vi "Write 16bit Wave.vi"() -> ()   [LabVIEW 2020]
uses:
  <vilib>/Analysis/NI_AALBase.lvlib
panel:
  out "16bit integer":i16[](array[numeric])
  # "ssh_init: Network error: Cannot assign requested address"
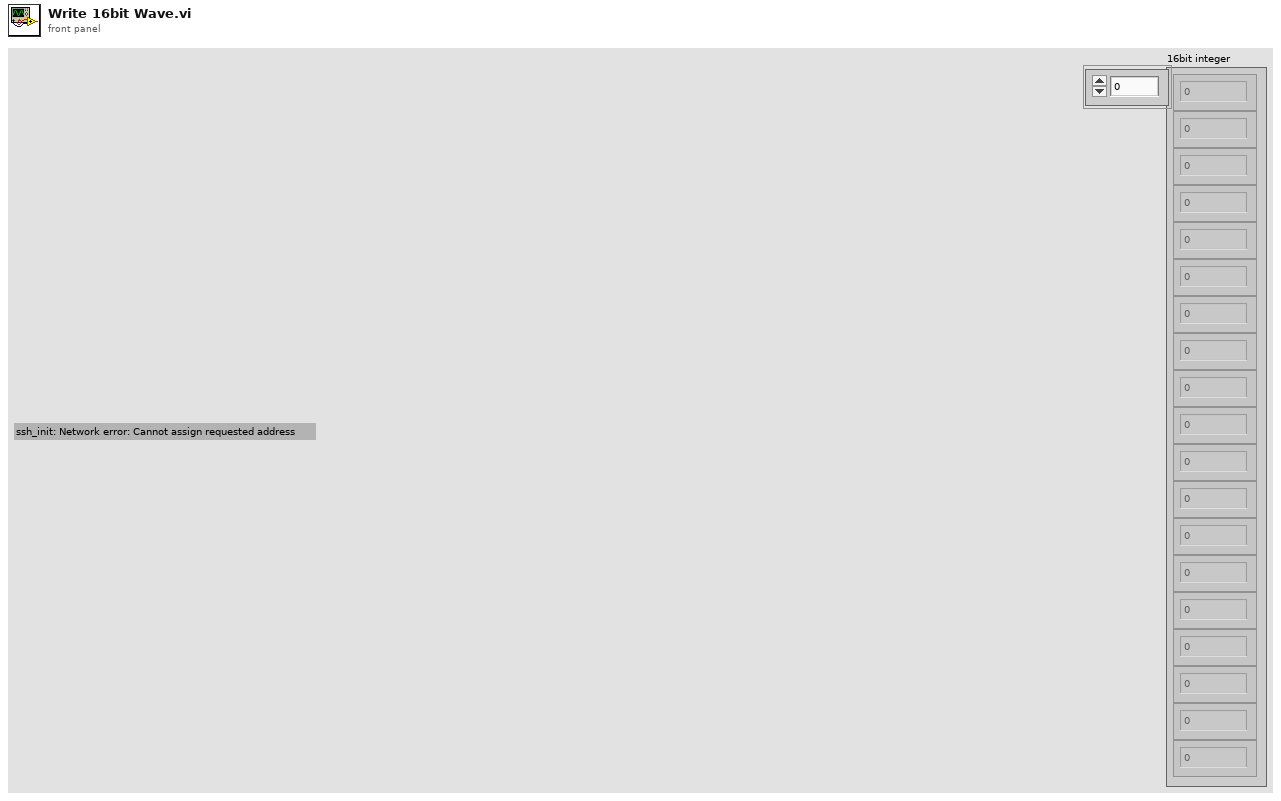
[diagram p1: front panel]
types:
  T1 = enum16{"big-endian, network order", "native, host order", "little-endian"}
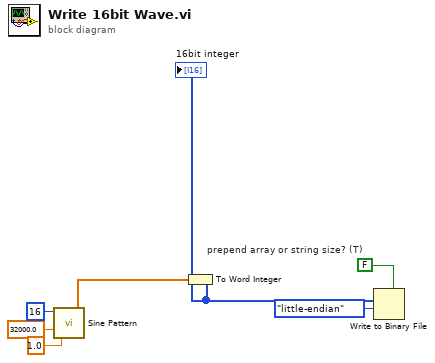
[diagram p0: block diagram]
diagram:
  w2 = FALSE  # prepend array or string size? (T)
  n1 = call <vilib>:"Sine Pattern.vi"("cycles"=1.0, "amplitude"=32000.0, "samples"=16) -> ("Sinusoidal Pattern"=w4:dbl[])  [unwired: 1 in, 1 out]
  n2 = To Word Integer(number=w4) -> (16bit integer=w3:i16[])
  "16bit integer" <- w3
  n3 = Write to Binary File(data=w3, 5:w2, 9:T1."little-endian" ("byte order (0:big-endian, network order)")) -> ()  [unwired: 3 in, 3 out]
